vi "SVPO Analog Tacho Process (1 Ch DBL Array).vi"(0 "analog tacho signal":dbl[](array[numeric]), 2 "reset? (F)":bool, 5 "sampling rate [Hz]":dbl=1.0, 7 "threshold":dbl format="%.2f", 9 "pulse/revolution (1)":i32=1, 11 "hysteresis (0)":dbl format="%.2f", 12 "pulse width (2)":i32=2, 13 "slope (Rising)":u16(ring) items=["Rising", "Falling"]) -> (4 "speed position info":T1, 6 "current speed [RPM]":dbl)   [LabVIEW 2017, in "SoundVib_TachProcess.lvlib"]
doc: "Locates tachometer pulse positions in analog tachometer signals using the number of generated pulses per revolution, the pulse width, and the arrival edge of the tachometer pulse. Use this VI on embedded targets that have limited computational resources. Wire data to the <B>analog tacho signal</B> input to determine the polymorphic instance to use or manually select the instance."
uses:
  <vilib>/addons/Sound and Vibration/Order Analysis/Tach Process/SoundVib_TachProcess.lvlib
  <vilib>/addons/Sound and Vibration/Order Analysis/Misc/OAT Position Info.ctl
  <vilib>/addons/Sound and Vibration/Order Analysis/Tach Process/SubVIs/oa_Convert Pulse Positions to Speed (No State).vi
  <vilib>/addons/Sound and Vibration/Order Analysis/Tach Process/SubVIs/sv_Edge Detection (1 Tach) with IC.vi
  <vilib>/addons/Sound and Vibration/Order Analysis/Tach Process/SubVIs/oa_Analog Tacho Hysteresis(1 Channel) with IC.vi
  <vilib>/addons/_NISVFA/_Shared subVIs/Common/SV Buffer Array (No State) (DBL).vi
  <vilib>/addons/Sound and Vibration/Order Analysis/Tach Process/SubVIs/OAT Cross Point Detection.vi
  <vilib>/addons/_NISVFA/_Shared subVIs/Common/svc_Get Array Subset (Index).vi
  <vilib>/Analysis/8numeric.llb/Threshold Detector.vi
  <vilib>/addons/_NISVFA/_Shared subVIs/Common/svc_Coerce Index and Length.vi
  <vilib>/addons/_NISVFA/_Shared subVIs/Common/svc_Conditional Merge Error.vi
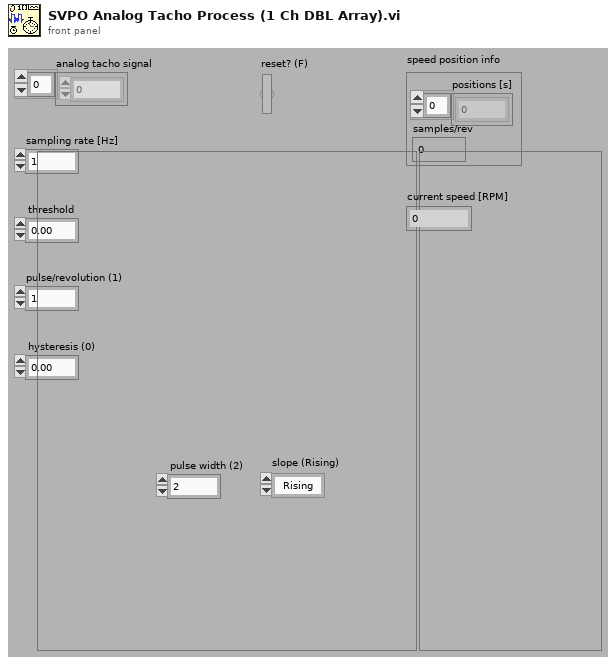
[diagram p1: front panel]
types:
  T1 = typedef "OAT Position Info.ctl" = cluster{"positions [s]":dbl[], "samples/rev":dbl}
  T2 = typedef "svc_Analog Tacho State.ctl" = cluster{"hysteresis state":dbl, "edge detection state":cluster{"x[n]":dbl[], "size":dbl}, "pulse to speed state":cluster{"pulse positions":dbl[], "elapsed time":dbl}}
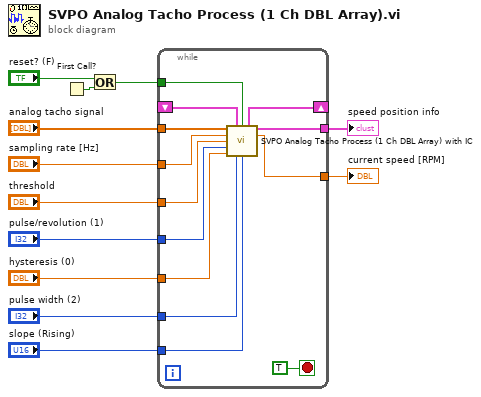
[diagram p0: block diagram]
diagram:
  n1 = First Call?() -> (First Call?: T/F=w11:bool)
  n2 = Or(x="reset? (F)", y=w11) -> (x .or. y?=w10:bool)
  n3 = while {
    tunnel: w10 -> [w25]
    tunnel: "analog tacho signal" -> [w24]
    tunnel: "hysteresis (0)" -> [w23]
    tunnel: "sampling rate [Hz]" -> [w22]
    tunnel: "threshold" -> [w21]
    tunnel: "slope (Rising)" -> [w20]
    tunnel: "pulse width (2)" -> [w19]
    tunnel: "pulse/revolution (1)" -> [w18]
    tunnel: [w17] -> w2
    tunnel: [w16] -> w1
    shift-right: [w14] -> _
    shift-left: _ -> [w13]
    stop <- TRUE stop-if-true
    n4 = call <vilib>:"SVPO Analog Tacho Process (1 Ch DBL Array) with IC.vi"("analog tacho signal"=w24, "initial conditions"=w13, "reset? (F)"=w25, "sampling rate [Hz]"=w22, "threshold"=w21, "pulse/revolution (1)"=w18, "hysteresis (0)"=w23, "pulse width (2)"=w19, "slope (Rising)"=w20) -> ("final conditions"=w14:T2, "speed position info"=w17:T1, "current speed [RPM]"=w16:dbl)  [unwired: 4 in]
  }
  "speed position info" <- w2
  "current speed [RPM]" <- w1
